vi "GetSensorByID.vi"(4 "Sensor ID":i32) -> (1 "Sensor Out":T1)   [LabVIEW 2014]
uses:
  SensorData.ctl
  navXPacket.ctl
  EncoderPacket.ctl
  PotentiometerPacket.ctl
  distanceSensorPacket.ctl
  switchPacket.ctl
  SensorType.ctl
  SensorStatus.ctl
  Global Data.vi
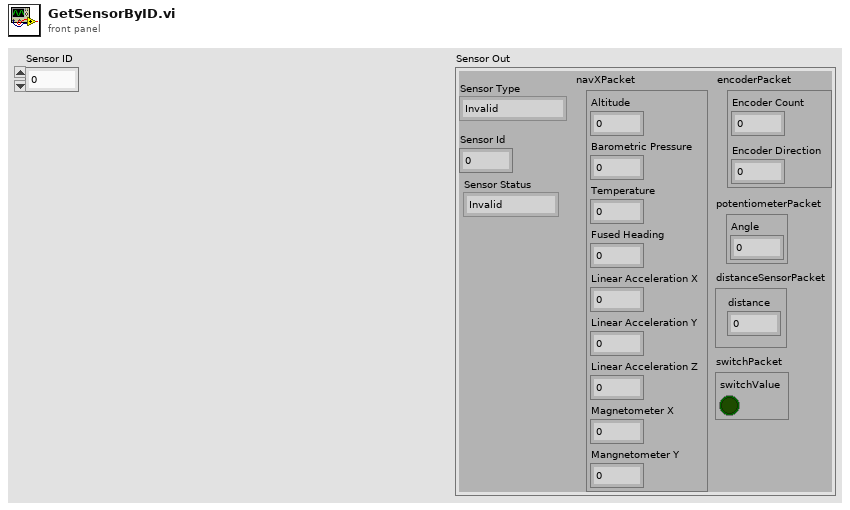
[diagram p1: front panel]
types:
  T1 = typedef "SensorData.ctl" = cluster{"Sensor Id":dbl, "navXPacket":T2, "encoderPacket":T3, "potentiometerPacket":T4, "distanceSensorPacket":T5, "switchPacket":T6, "Sensor Type":T7, "Sensor Status":T8}
  T2 = typedef "navXPacket.ctl" = cluster{"Altitude":dbl, "Barometric Pressure":dbl, "Fused Heading":dbl, "Linear Acceleration Y":dbl, "Linear Acceleration X":dbl, "Temperature":dbl, "Mangnetometer Y":dbl, "Magnetometer X":dbl, "Linear Acceleration Z":dbl}
  T3 = typedef "EncoderPacket.ctl" = cluster{"Encoder Count":dbl, "Encoder Direction":dbl}
  T4 = typedef "PotentiometerPacket.ctl" = cluster{"Angle":dbl}
  T5 = typedef "distanceSensorPacket.ctl" = cluster{"distance":dbl}
  T6 = typedef "switchPacket.ctl" = cluster{"switchValue":bool}
  T7 = typedef "SensorType.ctl" = enum16{"Invalid", "NavX", "Encoder", "Potentiometer", "Distance Sensor", "Switch"}
  T8 = typedef "SensorStatus.ctl" = enum16{"Invalid", "Operational", "Error occurred"}
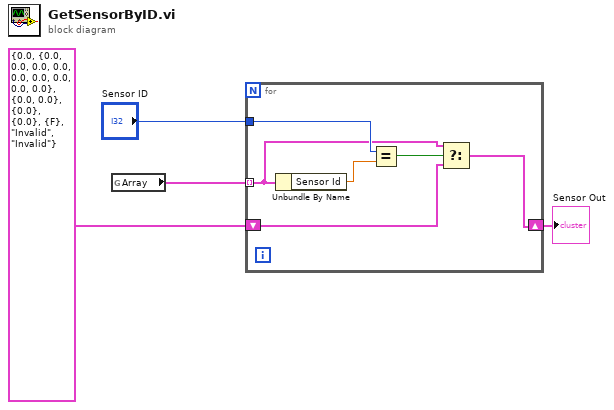
[diagram p0: block diagram]
diagram:
  n1 = global read "Global Data.vi" "Array"() -> (w3:T1[])
  n2 = for {
    tunnel: "Sensor ID" -> [w9]
    tunnel: w3 -> [w7] mode=indexing
    shift-right: [w5] -> w1
    shift-left: T1 {"Sensor Id"=0.0, "navXPacket"={"Altitude"=0.0, "Barometric Pressure"=0.0, "Fused Heading"=0.0, "Linear Acceleration Y"=0.0, "Linear Acceleration X"=0.0, "Temperature"=0.0, "Mangnetometer Y"=0.0, "Magnetometer X"=0.0, "Linear Acceleration Z"=0.0}, "encoderPacket"={"Encoder Count"=0.0, "Encoder Direction"=0.0}, "potentiometerPacket"={"Angle"=0.0}, "distanceSensorPacket"={"distance"=0.0}, "switchPacket"={"switchValue"=FALSE}, "Sensor Type"=enum."Invalid", "Sensor Status"=enum."Invalid"} ("Sensor Data") -> [w6]
    n3 = Unbundle By Name(w7) -> ("Sensor Id"=w10:dbl)
    n4 = Equal?(x=w9, y=w10) -> (x = y?=w8:bool)
    n5 = Select(t=w7, s=w8, f=w6) -> (s? t:f=w5:T1)
  }
  "Sensor Out" <- w1
